vi "WriteCSV.vi"(7 "新規/追記":enum16{"新規", "追記"}(ring), 8 "Error In":errorcluster caption="エラー入力", 10 "2D文字列":string[][](array[string]), 11 "ファイルパス":path) -> (0 "Error Out":errorcluster caption="エラー出力")   [LabVIEW 2015]
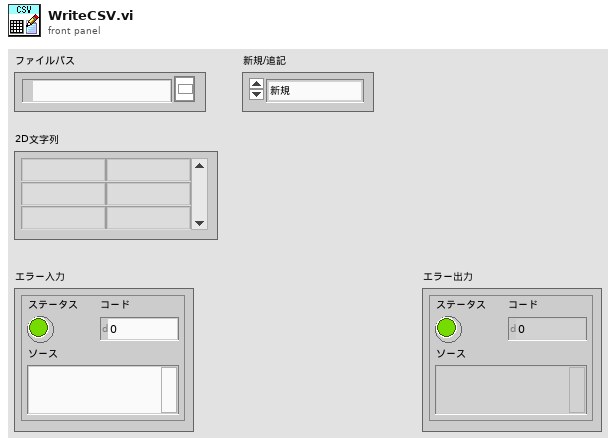
[diagram p1: front panel]
types:
  T1 = enum16{"open", "replace", "create", "open or create", "replace or create", "replace or create with confirmation"}
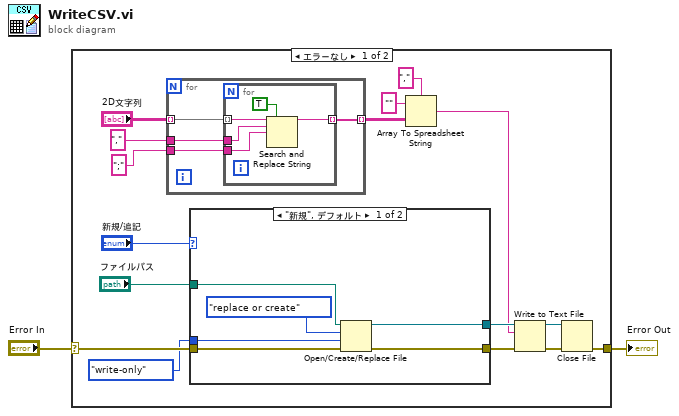
[diagram p0: block diagram]
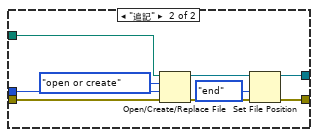
[diagram p2: hidden frame]
diagram:
  n1 = case shown="エラーなし" "Error In" {
    selector: "Error In" -> [w18 w43]
    tunnel: [w3 w43] -> w1
    frame No Error {
      n2 = for {
        tunnel: "2D文字列" -> [w22] mode=indexing
        tunnel: "," -> [w21]
        tunnel: ";" -> [w20]
        tunnel: [w19] -> w9 mode=indexing
        n3 = for {
          tunnel: w22 -> [w27] mode=indexing
          tunnel: w21 -> [w25]
          tunnel: w20 -> [w24]
          tunnel: [w23] -> w19 mode=indexing
          n4 = Search and Replace String(replace all?=TRUE ("すべて置換?（F）"), input string=w27, search string=w25, replace string=w24) -> (result string=w23:string)  [unwired: 4 in, 3 out]
        }
      }
      n5 = case shown="\"新規\", デフォルト" "新規/追記" {
        tunnel: w18 -> [w33 w42]
        tunnel: "ファイルパス" -> [w32 w39]
        tunnel: enum16{"read/write", "read-only", "write-only"}."write-only" ("アクセス （0:read/write）") -> [w30 w41]
        tunnel: [w29 w35] -> w10
        tunnel: [w28 w34] -> w11
        frame "新規", Default {
          n6 = Open/Create/Replace File(file path (use dialog)=w32, error in=w33, operation (0:open)=T1."replace or create" ("操作（0:open）"), access (0:read/write)=w30) -> (refnum out=w29:refnum<file>, error out=w28:errorcluster)  [unwired: 2 in, 1 out]
        }
        frame "追記" {
          n7 = Open/Create/Replace File(file path (use dialog)=w39, error in=w42, operation (0:open)=T1."open or create" ("操作（0:open）"), access (0:read/write)=w41) -> (refnum out=w38:refnum<file>, error out=w37:errorcluster)  [unwired: 2 in, 1 out]
          n8 = Set File Position(refnum=w38, from (0:start)=enum16{"start", "end", "current"}."end" ("基点（0:start）"), error in=w37) -> (refnum out=w35:refnum<file>, error out=w34:errorcluster)  [unwired: 1 in]
        }
      }
      n9 = Array To Spreadsheet String(delimiter (Tab)="," ("デリミタ（タブ）"), array=w9, 3:"" ("形式文字列")) -> (spreadsheet string=w6:string)
      n10 = Write to Text File(file (use dialog)=w10, text=w6, error in=w11) -> (refnum out=w4:refnum<file>, error out=w5:errorcluster)  [unwired: 1 in, 1 out]
      n11 = Close File(refnum=w4, error in=w5) -> (error out=w3:errorcluster)  [unwired: 1 out]
    }
    frame Error {
    }
  }
  "Error Out" <- w1
